vi "setDAQ.vi"(8 "error in (no error)":errorcluster, 10 "setDAQ":T1[](array[typedef]) {"AI.Coupling" items=["AC"=10045, "DC"=10050, "GND"=10066]}, 11 "Instrument.Lockin in":refnum<class "Instrument.Lockin.lvclass">) -> (0 "error out":errorcluster, 3 "Instrument.Lockin out":refnum<class "Instrument.Lockin.lvclass">)   [LabVIEW 2019, in "Instrument.Lockin.lvclass"]
doc: "API to configure AO.\n\nIf address=\"\", this API reads from localhost\nIf address is remote lockin, you need to add this computer to allowed whitelist on the lockin computer you are trying to access."
uses:
  Instrument.Lockin.lvclass
  C:/Program Files (x86)/National Instruments/LabVIEW 2019/user.lib/LevyLab/Levylab Instruments/SMOs/Instrument/Instrument.lvclass
  Instrument UI.Lockin/Typedefs/Device Configuration--Cluster.ctl
  Instrument.DAQ/Typedefs/446xAO-enum.ctl
  Instrument.DAQ/Typedefs/446xAI-enum.ctl
  Instrument.DAQ/Typedefs/AI.coupling-enum.ctl
  Typedefs/API/Lockin.Commands--Enum.ctl
  <userlib>/LevyLab/Levylab Instruments/SMOs/Instrument/Instrument.lvclass/Instrument.ctl
  e567dc32-cf46-45f2-a808-c6ffdf28405d.vi
  e567dc32-cf46-45f2-a808-c6ffdf28405d.vi/aaeddb97-d750-4ecb-80ee-da912f024880.vi
  e567dc32-cf46-45f2-a808-c6ffdf28405d.vi/aaeddb97-d750-4ecb-80ee-da912f024880.vi/ea1e7395-839e-415e-b03f-283a8998f0b8.vi
  <userlib>/LevyLab/Levylab Instruments/SMOs/Instrument/API/Send and Receive.vi
  e567dc32-cf46-45f2-a808-c6ffdf28405d.vi/aaeddb97-d750-4ecb-80ee-da912f024880.vi/ea1e7395-839e-415e-b03f-283a8998f0b8.vi/7f138455-d171-4de4-916d-73dcf11e926b.vi
  e567dc32-cf46-45f2-a808-c6ffdf28405d.vi/aaeddb97-d750-4ecb-80ee-da912f024880.vi/ea1e7395-839e-415e-b03f-283a8998f0b8.vi/b3694b7c-cd28-4962-97ae-72c56d45f0dd.vi
  <userlib>/LevyLab/Levylab Instruments/SMOs/Instrument/API/Enum to String.vi
  <userlib>/LevyLab/Levylab Instruments/SMOs/RemoteControl/API/Send and Receive.vi
  <vilib>/Utility/Data Type/Get Type Information.vi
  <vilib>/JDP Science/JSONtext/JSON text to Variant.vi
  <vilib>/JDP Science/JSONtext/LVClass Serializer/JSONtext LVClass Serializer.lvclass
  Instrument.DAQ/Instrument.DAQ.lvclass
  Instrument UI.Lockin/Instrument UI.Lockin.lvclass
panel:
  # "Device"
  # "AI.Ch"
  # "AI.Range"
  # "AI.Coupling"
  # "AO.Ch"
  # "AO.Range"
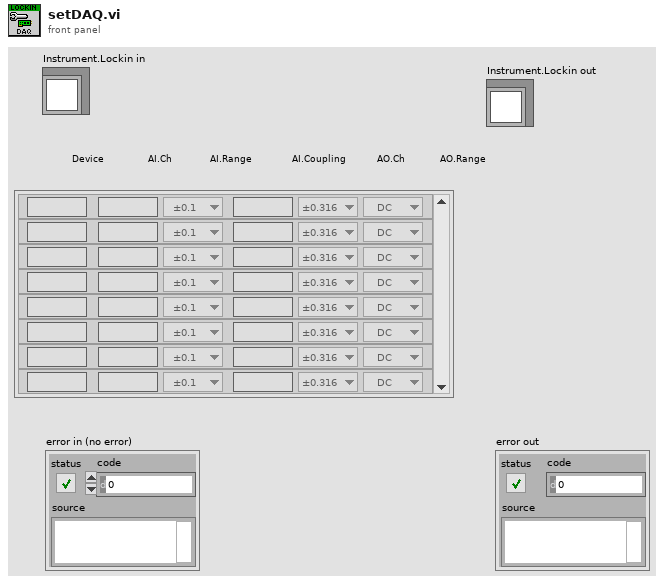
[diagram p1: front panel]
types:
  T1 = typedef "Instrument UI.Lockin.lvclass/Device Configuration--Cluster.ctl" = cluster{"Device":string, "AO.Ch":string, "AO.Range":T2, "AI.Ch":string, "AI.Range":T3, "AI.Coupling":T4}
  T2 = typedef "Instrument.DAQ.lvclass/446xAO-enum.ctl" = enum16{"±0.1", "±1.0", "±10.0"}
  T3 = typedef "Instrument.DAQ.lvclass/446xAI-enum.ctl" = enum16{"±0.316", "±1.00", "±3.16", "±10.0", "±31.6", "±42.4"}
  T4 = typedef "Instrument.DAQ.lvclass/AI.coupling-enum.ctl" = u16
  T5 = typedef "Instrument.Lockin.lvclass/Lockin.Commands--Enum.ctl" = enum16{"setAO", "setAO_Amplitude", "setAO_DC", "setAO_Frequency", "setAO_Phase", "setAO_Function", "setAO_I+", "setREF", "setREF_Frequency", "setREF_Phase", "setREF_TC", "setREF_Roll-Off", "setDAQ", "setSampling", "setOffset", "setState", "getState", "getAO", "getAI", "getResults", "getSampling", "getAOconfig", "getREFconfig", "setInputGain", "setOutputGain", "getInputGain", "getOutputGain", "setSamplingMode", "getSamplingMode", "setSweep", "getStatus", "getSweepResults", "getSweepWaveforms", "startSweep", "stopSweep", "setAUX", "getAUX", "getRefreshTime"}
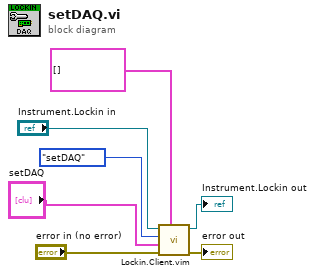
[diagram p0: block diagram]
diagram:
  n1 = call "Lockin.Client.vim"("Data Out type"=T1[] [] ("setDAQ"), "error in (no error)"="error in (no error)", "Data"="setDAQ", "Command"=Lockin.Commands--Enum."setDAQ", "Instrument.Lockin in"="Instrument.Lockin in") -> ("error out"=→"error out":errorcluster, "Instrument.Lockin out"=→"Instrument.Lockin out":refnum<class "Instrument.Lockin.lvclass">)  [unwired: 4 in, 1 out]
